vi "Delete String Array Element.vi"(10 "Element to Delete":string, 11 "Array in":string[](array[string])) -> (2 "Found and Deleted":bool, 3 "Array out":string[](array[string]))   [LabVIEW 2022 SP3, in "Wordle Engine.lvlib"]
uses:
  Wordle Engine.lvlib
  34fb09ad-82f2-4cc4-b24e-fe1593a329b2.vi
  <vilib>/Comparison/Equal/Equal Functor/Equal Functor.lvclass
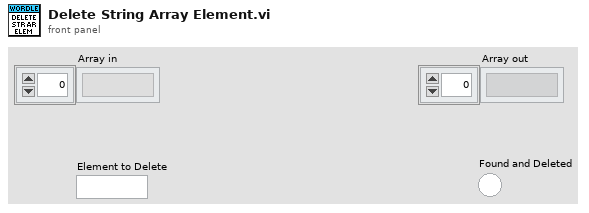
[diagram p1: front panel]
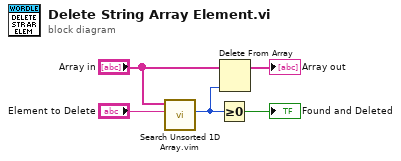
[diagram p0: block diagram]
diagram:
  n1 = call "Search Unsorted 1D Array.vim"("element"="Element to Delete", "unsorted 1D array"="Array in") -> ("index of element"=w2:i32)  [unwired: 9 in]
  n2 = Greater Or Equal To 0?(x=w2) -> (x >= 0?=→"Found and Deleted":bool)
  n3 = Delete From Array(array="Array in", index=w2) -> (array with subset deleted=→"Array out":string[])  [unwired: 1 in, 1 out]
